vi "FFT_DAS_Acq&Graph Voltage-Int Clk-SW Trig Restarts.vi"() -> ()   [LabVIEW 2010]
doc: "I. Description:\nThis example demonstrates how to acquire a finite amount of data (waveform) using the DAQ device's internal clock, each time a SW trigger is initiated. The SW trigger in this case is a simple boolean button. Additionally, the example shows how to efficiently restart the task therefore running at optimal speed.\n\nII. Instructions for Running:\n1. Select the physical channel to correspond to where your signal is input on the DAQ device.\n2. Enter the minimum and maximum voltages.\nNote: For better accuracy try to match the input range to the expected voltage level of the measured signal.\n3. Select the number of samples to acquire.\n4. Set the rate of the acquisition\nNote: The rate should be AT LEAST twice as fast as the maximum frequency component of the signal being acquired.\n5. Each time you want a finite block of data to be returned press the Acquire New Set of Data boolean control.\n\nIII. Block Diagram Steps:\n1. Create an analog input voltage channel(s)\n2. Set the rate for the sample clock. Additionally, define the sample mode to be finite and set the number of samples to be acquired per channel.\n3. Commit the settings into hardware by using the DAQmx Control Task VI. This allows for very efficient restarts\n4. Start acquiring data\n5. Use the Read VI to measure multiple samples from N Channels on the device. Set a timeout so an error is returned if the samples are not returned in the specified time limit\n6. Stop the task.\n5. Call the Clear Task VI to clear the Task after the acquisition is complete.\n6. Use the popup dialog box to display an error if any.\n \nIV. I/O Connections Overview:\nMake sure your signal input terminal matches the Physical Channel I/O Control. For further connection information, refer to your hardware reference manual."
uses:
  <vilib>/Utility/error.llb/DialogType.ctl
  <vilib>/Platform/TimedLoop/XDataNode/XDataNode.xnode
  <vilib>/Platform/TimedLoop/XDataNode/timing_clust.ctl
  <vilib>/Platform/TimedLoop/XDataNode/nitl_modes.ctl
  <vilib>/Platform/TimedLoop/XDataNode/wakeup.ctl
  <vilib>/DAQmx/read.llb/DAQmx Read.vi
  <vilib>/DAQmx/create/channels.llb/DAQmx Create Virtual Channel.vi
  <vilib>/DAQmx/configure/timing.llb/DAQmx Timing.vi
  <vilib>/daqmx/miscellaneous.llb/DAQmx Fill In Error Info.vi
  <vilib>/Platform/TimedLoop/XDataNode/XDNodeRunTimeDep.lvlib
panel:
  in  "device in":tag
  in  "Acquire New Set of Data\n(Software Trigger)":bool
  in  "stop":bool
  in  "Maximum Value":dbl=10.0 format="%0.2f"
  in  "Minimum Value":dbl=-10.0 format="%0.2f"
  in  "Physical Channel":tag="Dev1/ai0"
  in  "Rate":dbl=50000.0 caption="Sample Rate (Hz)" format="%0.2f"
  in  "Samples per Channel":i32=2048
  out "Measurement":waveform(dbl)[](graph)
  # "For instructions, select Help>>Show Context Help"
  # "Channel Parameters"
  # "Timing Parameters"
  # "A new set of points is acquired every time\nyou press this boolean button."
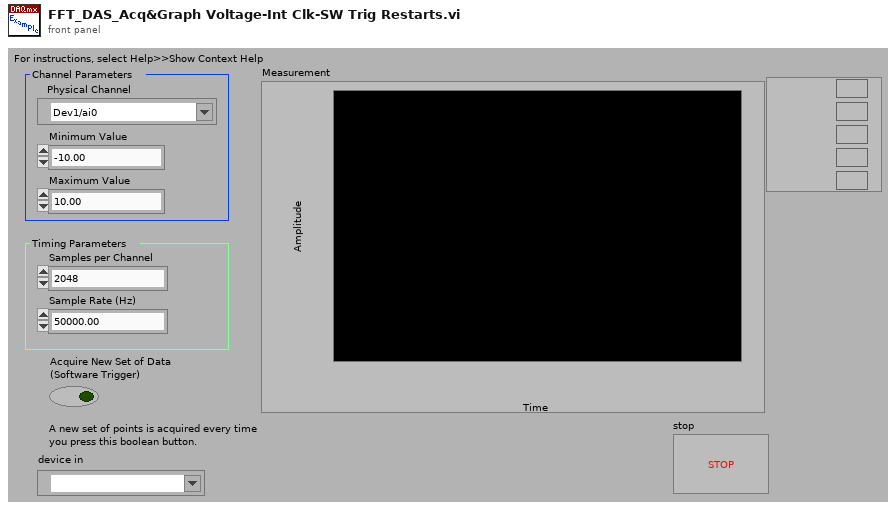
[diagram p1: front panel]
types:
  T1 = typedef "DialogType.ctl" = u16
  T2 = typedef "XDNodeRunTimeDep.lvlib/timing_clust.ctl" = cluster{"Expected End [f-1]":u64, "Actual End [f-1]":u64, "Finished Late? [f-1]":bool, "Expected End [i-1]":u64, "Actual End [i-1]":u64, "Finished Late? [i-1]":bool, "Expected Start [i]":u64, "Actual Start [i]":u64, "Expected Start [f]":u64, "Actual Start [f]":u64, "Source Name":string, "Structure Name":string, "Period":i64, "Deadline":i64, "Offset":i64, "Start":i64, "Priority":i32, "Timeout":i32, "Mode":T3, "Wakeup Reason":T4, "Error":errorcluster, "Source Type":string, "Secondary Source Type":string, "Global End Time":u64, "Global Start Time":u64, "Frame Duration":u64, "Iteration Duration":u64, "Assigned CPU":i32, "I/O Scan Engine Mode":u32}
  T3 = typedef "XDNodeRunTimeDep.lvlib/nitl_modes.ctl" = enum32{"No Change", "Process missed periods, maintain original phase", "Discard missed periods, maintain original phase", "Process missed periods, ignore original phase", "Discard missed periods, ignore original phase"}
  T4 = typedef "XDNodeRunTimeDep.lvlib/wakeup.ctl" = enum32{"Normal", "Aborted", "Asynchronous wakeup", "Timing source error", "Timed loop error", "Timeout"}
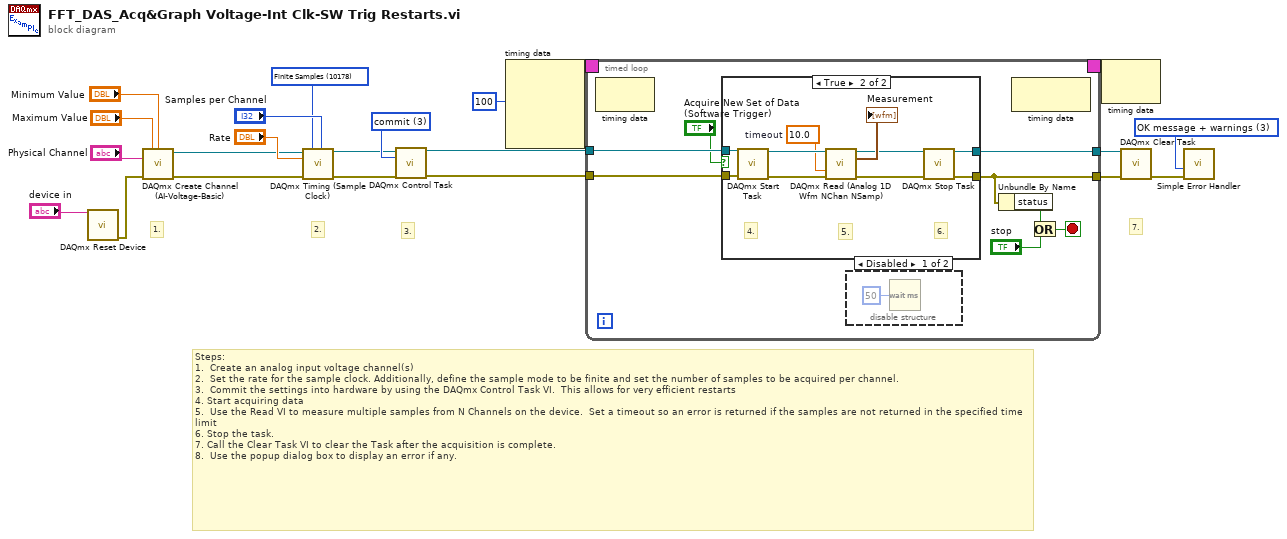
[diagram p0: block diagram]
diagram:
  w12 = 3 items=["verify"=2, "reserve"=4, "commit"=3, "unreserve"=5, "abort"=6] ("action")
  w13 = T1 3 items=["no dialog", "OK message", "continue or stop message", "OK message + warnings", "continue/stop + warnings"] ("type of dialog (OK msg:1)")
  w14 = 10178 items=["Finite Samples"=10178, "Continuous Samples"=10123] ("sample mode")
  # "7."
  # "Steps: \n1.  Create an analog input voltage channel(s)\n2.  Set the rate for the sample clock. Additionally, define the sample mode to be finite and set the number of samples to be acquired per channel.\n3.  Commit the settings into hardware by using the DAQmx Control Task VI.  This allows for very efficient restarts\n4. Start acquiring data\n5.  Use the Read VI to measure multiple samples from N Channels on the device.  Set a timeout so an error is returned if the samples are not returned in the specified time limit\n6. Stop the task.\n7. Call the Clear Task VI to clear the Task after the acquisition is complete.\n8.  Use the popup dialog box to display an error if any."
  # "3."
  # "2."
  # "1."
  n1 = call <vilib>:"DAQmx Reset Device.vi"("device in"="device in") -> ("error out"=w4:errorcluster)  [unwired: 14 in]
  n2 = call-poly <vilib>:"DAQmx Create Channel (AI-Voltage-Basic).vi"("maximum value"="Maximum Value", "minimum value"="Minimum Value", "physical channels"="Physical Channel", "error in"=w4) -> ("task out"=w16:refnum<k21>, "error out"=w20:errorcluster)  [unwired: 10 in]
  n3 = call-poly <vilib>:"DAQmx Timing (Sample Clock).vi"("task/channels in"=w16, "sample mode"=w14, "samples per channel"="Samples per Channel", "rate"="Rate", "error in"=w20) -> ("task out"=w11:refnum<k21>, "error out"=w10:errorcluster)  [unwired: 9 in]
  n4 = call <vilib>:"DAQmx Control Task.vi"("task/channels in"=w11, "action"=w12, "error in"=w10) -> ("task out"=w9:refnum<k21>, "error out"=w8:errorcluster)  [unwired: 11 in]
  n5 = node-c288(i64 100 ("Period")) -> (w3:T2)  [unwired: 3 in]
  n6 = timed-loop {
    tunnel: w9 -> [w30]
    tunnel: w8 -> [w29]
    tunnel: [w28] -> w7
    tunnel: [w26] -> w6
    timing: w3 -> [_]
    timing-out: [_] -> w2
    stop <- w23 stop-if-true
    n7 = node-c288() -> ()  [unwired: 1 in, 1 out]
    n8 = case shown="True" "Acquire New Set of Data\n(Software Trigger)" {
      tunnel: w30 -> [w35 w41]
      tunnel: w29 -> [w34 w40]
      tunnel: [w35 w37] -> w28
      tunnel: [w34 w36] -> w26
      frame False {
      }
      frame True {
        w42 = 10.0  # timeout
        # "6."
        # "5."
        # "4."
        n9 = call <vilib>:"DAQmx Start Task.vi"("task/channels in"=w41, "error in"=w40) -> ("task out"=w44:refnum<k21>, "error out"=w45:errorcluster)  [unwired: 12 in]
        n10 = call-poly <vilib>:"DAQmx Read (Analog 1D Wfm NChan NSamp).vi"("task/channels in"=w44, "timeout"=w42, "error in"=w45) -> ("task out"=w39:refnum<k21>, "data"=→"Measurement":waveform(dbl)[], "error out"=w38:errorcluster)  [unwired: 10 in]
        n11 = call <vilib>:"DAQmx Stop Task.vi"("task/channels in"=w39, "error in"=w38) -> ("task out"=w37:refnum<k21>, "error out"=w36:errorcluster)  [unwired: 12 in]
      }
    }
    n12 = disable-structure shown="Disabled" {
      frame Disabled {
        n13 = Wait (ms)(milliseconds to wait=u32 50) -> ()  [unwired: 1 out]
      }
      frame Enabled {
      }
    }
    n14 = Unbundle By Name(w26) -> ("status"=w25:bool)
    n15 = node-c288() -> ()  [unwired: 1 in, 1 out]
    n16 = Or(x=w25, y="stop") -> (x .or. y?=w23:bool)
  }
  n17 = node-c288(w2) -> ()  [unwired: 1 out]
  n18 = call <vilib>:"DAQmx Clear Task.vi"("task in"=w7, "error in"=w6) -> ("error out"=w18:errorcluster)  [unwired: 13 in]
  n19 = call <vilib>:"Simple Error Handler.vi"("type of dialog (OK msg:1)"=w13, "error in (no error)"=w18) -> ()  [unwired: 3 in, 5 out]
